vi "Read Module Name.vi"(8 "error in (no error)":errorcluster, 11 "Rename in":refnum<class "Rename.lvclass">) -> (0 "error out":errorcluster, 2 "Module Name":string, 3 "Rename out":refnum<class "Rename.lvclass">)   [LabVIEW 2015, in "Generic Module Library.lvlib" / "Template G_Module.lvlib" / "Rename.lvclass"]
uses:
  Rename.lvclass
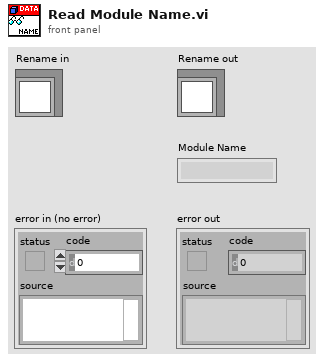
[diagram p1: front panel]
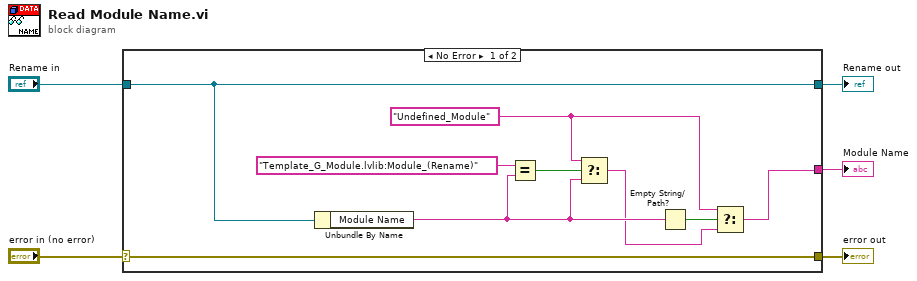
[diagram p0: block diagram]
diagram:
  n1 = case shown="No Error" "error in (no error)" {
    selector: "error in (no error)" -> [w14 w15]
    tunnel: [w14 w15] -> w4
    tunnel: [w13 w16] -> w2
    tunnel: "Rename in" -> [w13 w16]
    tunnel: [w6 _] -> w1
    frame No Error {
      w10 = "Undefined_Module"
      n2 = Unbundle By Name(w13) -> ("Module Name"=w8:string)
      n3 = Equal?(x="Template_G_Module.lvlib:Module_(Rename)", y=w8) -> (x = y?=w11:bool)
      n4 = Select(t=w10, s=w11, f=w8) -> (s? t:f=w7:string)
      n5 = Empty String/Path?(string/path=w8) -> (empty?=w9:bool)
      n6 = Select(t=w10, s=w9, f=w7) -> (s? t:f=w6:string)
    }
    frame Error {
    }
  }
  "error out" <- w4
  "Rename out" <- w2
  "Module Name" <- w1
